vi "GetPositionUm.vi"(8 "error in (no error)":errorcluster, 10 "Stage Label":string, 11 "Stage_MadCityLab in":refnum<class "Stage_MadCityLab.lvclass">) -> (0 "error out":errorcluster, 2 "Stage Position":dbl, 3 "Stage_MadCityLab out":refnum<class "Stage_MadCityLab.lvclass">)   [LabVIEW 2020, in "Stage_MadCityLab.lvlib" / "Stage_MadCityLab.lvclass"]
uses:
  Stage_MadCityLab.lvclass
  Dependency/Madlib.dll
  <vilib>/ActorFramework/Actor/Actor.lvclass
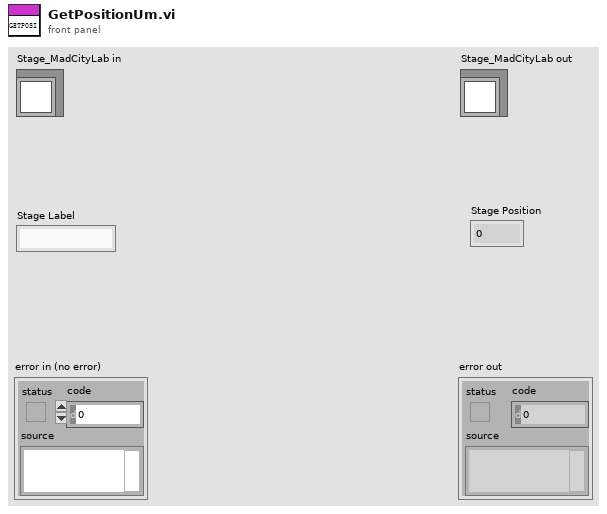
[diagram p1: front panel]
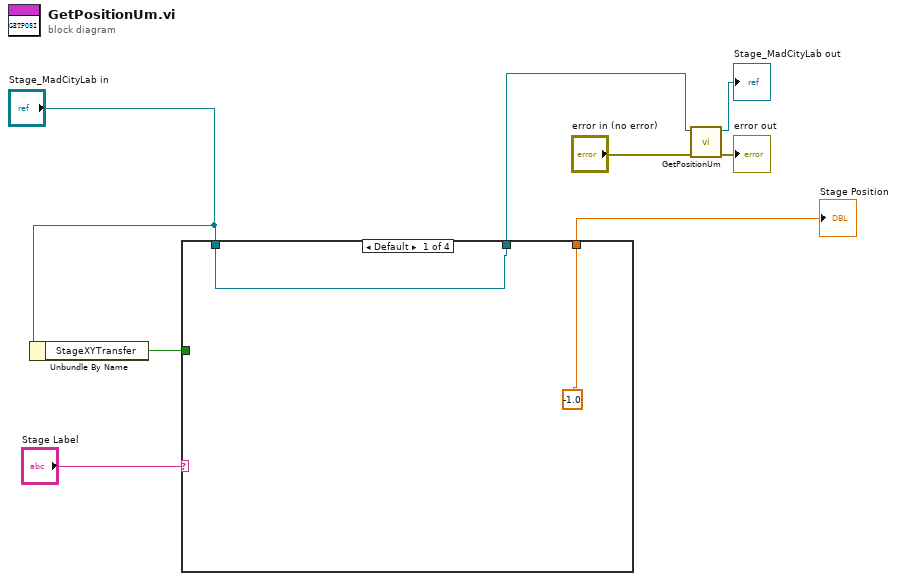
[diagram p0: block diagram]
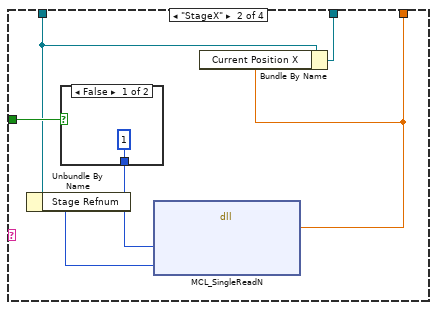
[diagram p2: hidden frame]
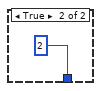
[diagram p3: hidden frame]
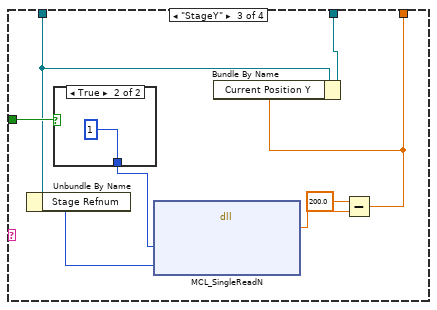
[diagram p4: hidden frame]
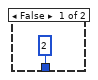
[diagram p5: hidden frame]
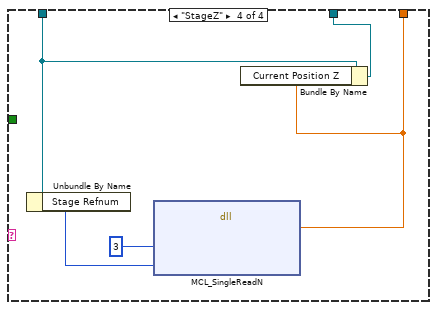
[diagram p6: hidden frame]
diagram:
  n1 = Unbundle By Name("Stage_MadCityLab in") -> ("StageXYTransfer"=w2:bool)
  n2 = case shown="Default" "Stage Label" {
    tunnel: "Stage_MadCityLab in" -> [w9 w12 w21 w30]
    tunnel: [-1.0 ("return type") w11 w19 w29] -> w4
    tunnel: w2 -> [_ w15 w25 _]
    tunnel: [w9 w13 w20 w31] -> w1
    frame Default {
    }
    frame "StageX" {
      n3 = Unbundle By Name(w12) -> ("Stage Refnum"=w16:i32)
      n4 = case shown="False" w15 {
        tunnel: [u32 1 ("axis") u32 2 ("axis")] -> w14
        frame False {
        }
        frame True {
        }
      }
      n5 = dll-call lib="E:/Development/DevHardSoftware/MicroscopyFramework/Model/Hardware Layer/Real Hardware/Stage_MadCityLab/Stage_MadCityLab/Dependency/Madlib.dll" fn="MCL_SingleReadN"("axis"=w14, "handle"=w16) -> ("return type"=w11:dbl)  [unwired: 5 in, 2 out]
      n6 = Bundle By Name(cluster=w12, "Current Position X"=w11) -> (w13:refnum<class "Stage_MadCityLab.lvclass">)
    }
    frame "StageY" {
      n7 = Unbundle By Name(w21) -> ("Stage Refnum"=w26:i32)
      n8 = case shown="True" w25 {
        tunnel: [u32 2 ("axis") u32 1 ("axis")] -> w24
        frame False {
        }
        frame True {
        }
      }
      n9 = dll-call lib="E:/Development/DevHardSoftware/MicroscopyFramework/Model/Hardware Layer/Real Hardware/Stage_MadCityLab/Stage_MadCityLab/Dependency/Madlib.dll" fn="MCL_SingleReadN"("axis"=w24, "handle"=w26) -> ("return type"=w23:dbl)  [unwired: 5 in, 2 out]
      n10 = Subtract(x=200.0, y=w23) -> (x-y=w19:dbl)
      n11 = Bundle By Name(cluster=w21, "Current Position Y"=w19) -> (w20:refnum<class "Stage_MadCityLab.lvclass">)
    }
    frame "StageZ" {
      n12 = Unbundle By Name(w30) -> ("Stage Refnum"=w33:i32)
      n13 = dll-call lib="E:/Development/DevHardSoftware/MicroscopyFramework/Model/Hardware Layer/Real Hardware/Stage_MadCityLab/Stage_MadCityLab/Dependency/Madlib.dll" fn="MCL_SingleReadN"("axis"=u32 3, "handle"=w33) -> ("return type"=w29:dbl)  [unwired: 5 in, 2 out]
      n14 = Bundle By Name(cluster=w30, "Current Position Z"=w29) -> (w31:refnum<class "Stage_MadCityLab.lvclass">)
    }
  }
  "Stage Position" <- w4
  n15 = call-parent "GetPositionUm.vi"("error in (no error)"="error in (no error)", "Stage in"=w1) -> ("error out"=→"error out":errorcluster, "Stage out"=→"Stage_MadCityLab out":refnum<class "Stage_MadCityLab.lvclass">)  [unwired: 7 in, 1 out]
